vi "SteeringManager_main.vi"(8 "Error in":errorcluster) -> (0 "Error Out":errorcluster)   [LabVIEW 2013]
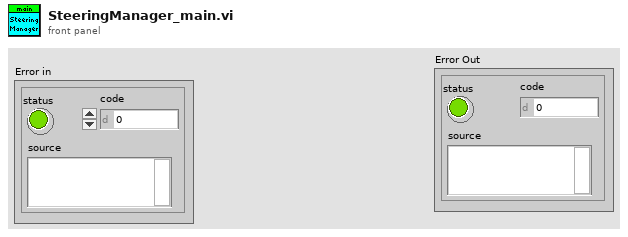
[diagram p1: front panel]
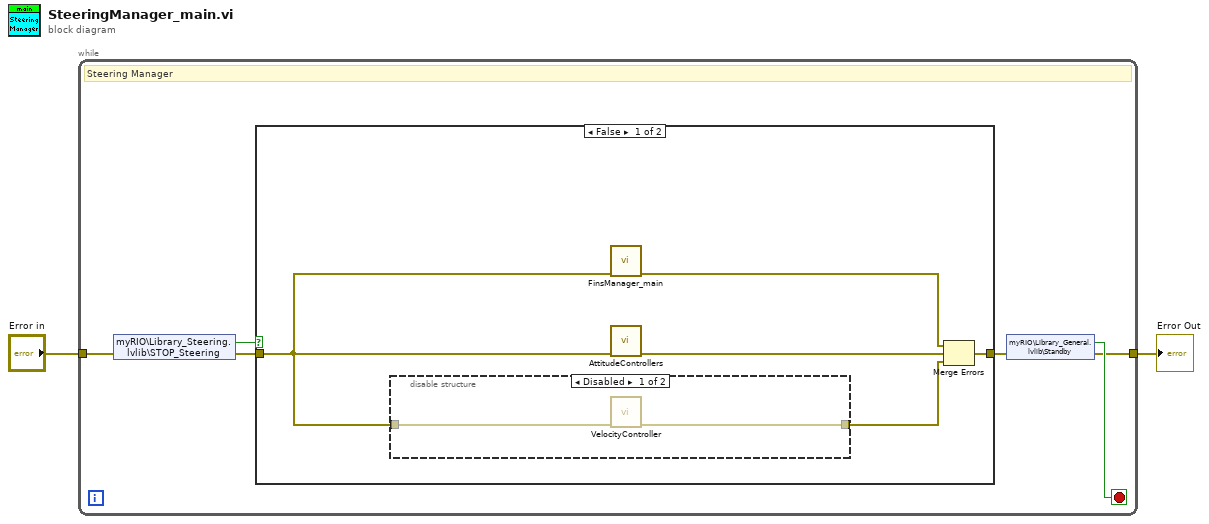
[diagram p0: block diagram]
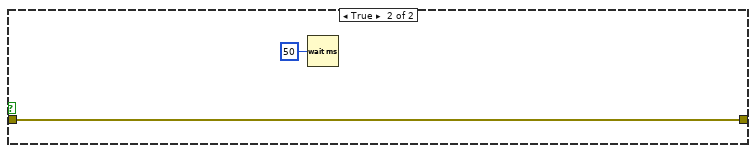
[diagram p3: hidden frame]
diagram:
  n1 = while {
    tunnel: "Error in" -> [w4]
    tunnel: [w6] -> w1
    stop <- w8 stop-if-true
    # "Steering Manager"
    n2 = shared-variable "myRIO\\Library_Steering.lvlib\\STOP_Steering"(error in=w4) -> (w7:bool, error out=w3:errorcluster)
    n3 = case shown="False" w7 {
      tunnel: w3 -> [w10 w17]
      tunnel: [w13 w17] -> w5
      frame False {
        n4 = disable-structure shown="Disabled" {
          disable-tunnel: w10 -> [w15 w16]
          disable-tunnel: [w14 w16] -> w9
          frame Disabled {
            n5 = call "VelocityController.vi"("error in (no error)"=w15) -> ("error out"=w14:errorcluster)  [unwired: 10 in]
          }
          frame Enabled {
          }
        }
        n6 = call "FinsManager_main.vi"("Error In"=w10) -> ("Error Out"=w12:errorcluster)  [unwired: 10 in]
        n7 = call "AttitudeControllers.vi"("error in (no error)"=w10) -> ("error out"=w11:errorcluster)  [unwired: 10 in]
        n8 = Merge Errors(w12, w11, w9) -> (w13:errorcluster)
      }
      frame True {
        n9 = Wait (ms)(milliseconds to wait=u32 50) -> ()  [unwired: 1 out]
      }
    }
    n10 = shared-variable "myRIO\\Library_General.lvlib\\Standby"(error in=w5) -> (w8:bool, error out=w6:errorcluster)
  }
  "Error Out" <- w1
